vi "HTTPS Server Test with BIO & TCPIP Nodes.vi"() -> ()   [LabVIEW 2013]
uses:
  SSL_Lib/SSL-Lib/Library Paths.ctl
  SSL_Lib/SSL/SSL_Mode.ctl
  SSL_Lib/SSL-Lib/SSL-Lib.lvclass
  SSL_Lib/SSL-Context/SSL-Context.lvclass
  SSL_Lib/SSL/SSL.lvclass
  SSL_Lib/BIO/BIO.lvclass
panel:
  out "Read bytes":string
  out "Numeric":i32
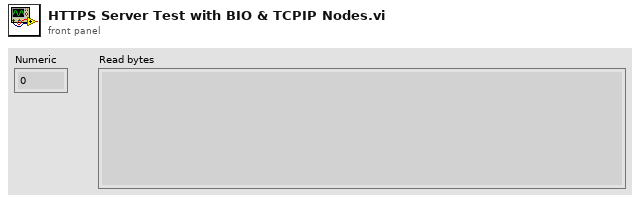
[diagram p1: front panel]
types:
  T1 = typedef "SSL_Lib.lvlib/SSL.lvclass/SSL_Mode.ctl" = i32
  T2 = typedef "SSL_Lib.lvlib/SSL-Lib.lvclass/Library Paths.ctl" = cluster{"SSL Library Path":path, "Crypto Library Path":path}
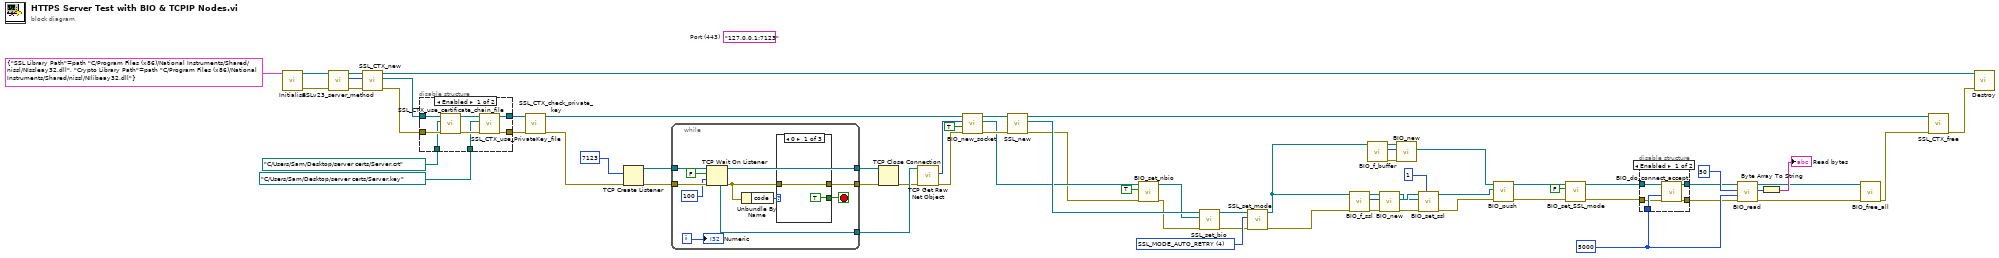
[diagram p0: block diagram]
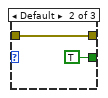
[diagram p3: hidden frame]
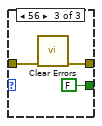
[diagram p4: hidden frame]
diagram:
  w37 = u32 5000 ("Timeout (10000ms)")
  (unwired) "127.0.0.1:7123"  # Port (443)
  w54 = T1 4 items=["None"=0, "SSL_MODE_ENABLE_PARTIAL_WRITE"=1, "SSL_MODE_ACCEPT_MOVING_WRITE_BUFFER"=2, "SSL_MODE_AUTO_RETRY"=4, "SSL_MODE_RELEASE_BUFFERS"=16, "SSL_MODE_SEND_FALLBACK_SCSV"=128] ("Mode")
  n1 = call "Initialise.vi"("Library Paths"=T2 {"SSL Library Path"=path "C:/Program Files (x86)/National Instruments/Shared/nissl/NIssleay32.dll", "Crypto Library Path"=path "C:/Program Files (x86)/National Instruments/Shared/nissl/NIlibeay32.dll"}) -> ("error out"=w63:errorcluster, "SSL-Lib out"=w67:refnum<class "SSL-Lib.lvclass">)  [unwired: 9 in]
  n2 = call "SSLv23_server_method.vi"("error in (no error)"=w63, "SSL-Lib in"=w67) -> ("error out"=w61:errorcluster, "*SSL_Method"=w66:u64, "SSL-Lib out"=w65:refnum<class "SSL-Lib.lvclass">)  [unwired: 7 in]
  n3 = call "SSL_CTX_new.vi"("error in (no error)"=w61, "*SSL_Method"=w66, "SSL-Lib in"=w65) -> ("error out"=w60:errorcluster, "SSL-Context out"=w59:refnum<class "SSL-Context.lvclass">, "SSL-Lib out"=w53:refnum<class "SSL-Lib.lvclass">)  [unwired: 6 in]
  n4 = disable-structure shown="Enabled" {
    disable-tunnel: w60 -> [w73 w76]
    disable-tunnel: w59 -> [w72 w77]
    disable-tunnel: [w71 w76] -> w58
    disable-tunnel: [w70 w77] -> w57
    disable-tunnel: path "C:/Users/Sam/Desktop/server certs/Server.crt" -> [w69 _]
    disable-tunnel: path "C:/Users/Sam/Desktop/server certs/Server.key" -> [w68 _]
    frame Enabled {
      n5 = call "SSL_CTX_use_certificate_chain_file.vi"("error in (no error)"=w73, "Certificate Chain File"=w69, "SSL-Context in"=w72) -> ("error out"=w75:errorcluster, "SSL-Context out"=w74:refnum<class "SSL-Context.lvclass">)  [unwired: 7 in]
      n6 = call "SSL_CTX_use_PrivateKey_file.vi"("error in (no error)"=w75, "PrivateKey File"=w68, "SSL-Context in"=w74) -> ("error out"=w71:errorcluster, "SSL-Context out"=w70:refnum<class "SSL-Context.lvclass">)  [unwired: 7 in]
    }
    frame Disabled {
    }
  }
  n7 = call "SSL_CTX_check_private_key.vi"("error in (no error)"=w58, "SSL-Context in"=w57) -> ("error out"=w45:errorcluster, "SSL-Context out"=w30:refnum<class "SSL-Context.lvclass">)  [unwired: 8 in]
  n8 = TCP Create Listener(8:w45, 10:u16 7123 ("port")) -> (0:w51:errorcluster, 3:w50:refnum<k5>)  [unwired: 3 in, 1 out]
  n9 = while {
    tunnel: w51 -> [w88]
    tunnel: w50 -> [w87]
    tunnel: [w86] -> w49
    tunnel: [w82] -> w48
    tunnel: [w85] -> w47
    i -> [w78]
    stop <- w81 stop-if-true
    n10 = TCP Wait On Listener(8:w88, 9:100 ("timeout ms (wait forever: -1)"), 10:FALSE ("resolve remote address (T)"), 11:w87) -> (0:w83:errorcluster, 3:w86:refnum<k5>, 4:w85:refnum<k5>)  [unwired: 2 out]
    n11 = Unbundle By Name(w83) -> ("code"=w84:i32)
    n12 = case shown="0" w84 {
      tunnel: w83 -> [w90 w92 w95]
      tunnel: [w90 w92 w94] -> w82
      tunnel: [TRUE TRUE FALSE] -> w81
      frame 0 {
      }
      frame Default {
      }
      frame 56 {
        n13 = call <vilib>:"Clear Errors.vi"("error in (no error)"=w95) -> ("error out"=w94:errorcluster)  [unwired: 6 in]
      }
    }
    "Numeric" <- w78
  }
  n14 = TCP Close Connection(connection ID=w49, error in (no error)=w48) -> (error out=w46:errorcluster)  [unwired: 1 in, 1 out]
  n15 = call <vilib>:"TCP Get Raw Net Object.vi"("error in (no error)"=w46, "connection ID"=w47) -> ("error out"=w33:errorcluster, "raw net object"=w32:u64)  [unwired: 7 in, 1 out]
  n16 = call "BIO_new_socket.vi"("error in (no error)"=w33, "Close on free? (T)"=TRUE, "fd"=w32, "SSL-Context in"=w30) -> ("error out"=w29:errorcluster, "Socket BIO out"=w26:refnum<class "BIO.lvclass">, "SSL-Context out"=w28:refnum<class "SSL-Context.lvclass">)  [unwired: 5 in]
  n17 = call "SSL_new.vi"("error in (no error)"=w29, "SSL-Context in"=w28) -> ("error out"=w23:errorcluster, "SSL out"=w27:refnum<class "SSL.lvclass">, "SSL-Context out"=w44:refnum<class "SSL-Context.lvclass">)  [unwired: 7 in]
  n18 = call "BIO_set_nbio.vi"("error in (no error)"=w23, "Non-Blocking?"=TRUE, "BIO in"=w26) -> ("error out"=w22:errorcluster, "BIO out"=w24:refnum<class "BIO.lvclass">)  [unwired: 7 in]
  n19 = call "SSL_set_bio.vi"("error in (no error)"=w22, "BIO"=w24, "SSL in"=w27) -> ("error out"=w21:errorcluster, "SSL out"=w25:refnum<class "SSL.lvclass">)  [unwired: 7 in]
  n20 = call "SSL_set_mode.vi"("error in (no error)"=w21, "Mode"=w54, "SSL in"=w25) -> ("error out"=w12:errorcluster, "SSL out"=w5:refnum<class "SSL.lvclass">)  [unwired: 7 in]
  n21 = call "BIO_f_ssl.vi"("error in (no error)"=w12, "SSL-Lib in"=w5) -> ("error out"=w17:errorcluster, "*BIO_Method"=w15:u64, "SSL-Lib out"=w16:refnum<class "SSL.lvclass">)  [unwired: 7 in]
  n22 = call "BIO_f_buffer.vi"("SSL-Lib in"=w5) -> ("error out"=w20:errorcluster, "*BIO_Method"=w18:u64, "SSL-Lib out"=w19:refnum<class "SSL.lvclass">)  [unwired: 8 in]
  n23 = call "BIO_new.vi"("error in (no error)"=w17, "*BIO_method"=w15, "SSL-Lib in"=w16) -> ("error out"=w14:errorcluster, "BIO out"=w13:refnum<class "BIO.lvclass">, "SSL-Lib out"=w11:refnum<class "SSL.lvclass">)  [unwired: 6 in]
  n24 = call "BIO_new.vi"("error in (no error)"=w20, "*BIO_method"=w18, "SSL-Lib in"=w19) -> ("BIO out"=w9:refnum<class "BIO.lvclass">)  [unwired: 6 in, 2 out]
  n25 = call "BIO_set_ssl.vi"("close flag"=1, "error in (no error)"=w14, "SSL in"=w11, "BIO in"=w13) -> ("error out"=w7:errorcluster, "BIO out"=w8:refnum<class "BIO.lvclass">)  [unwired: 6 in]
  n26 = call "BIO_push.vi"("error in (no error)"=w7, "New BIO"=w8, "BIO in"=w9) -> ("error out"=w6:errorcluster, "BIO out"=w3:refnum<class "BIO.lvclass">)  [unwired: 7 in]
  n27 = call "BIO_set_SSL_mode.vi"("error in (no error)"=w6, "Client?"=FALSE, "BIO in"=w3) -> ("error out"=w4:errorcluster, "BIO out"=w2:refnum<class "BIO.lvclass">)  [unwired: 7 in]
  n28 = disable-structure shown="Enabled" {
    disable-tunnel: w2 -> [w100 w102]
    disable-tunnel: w37 -> [w99 _]
    disable-tunnel: [w98 w102] -> w36
    disable-tunnel: [w97 w101] -> w35
    disable-tunnel: w4 -> [w96 w101]
    frame Enabled {
      n29 = call "BIO_do_connect_accept.vi"("error in (no error)"=w96, "Timeout (10000ms)"=w99, "BIO in"=w100) -> ("error out"=w97:errorcluster, "BIO out"=w98:refnum<class "BIO.lvclass">)  [unwired: 7 in]
    }
    frame Disabled {
    }
  }
  n30 = call "BIO_read.vi"("error in (no error)"=w35, "Timeout (10000ms)"=w37, "bytes to read"=50, "BIO in"=w36) -> ("error out"=w39:errorcluster, "Bytes read"=w41:u8[], "BIO out"=w34:refnum<class "BIO.lvclass">)  [unwired: 5 in]
  n31 = Byte Array To String(unsigned byte array=w41) -> (string=→"Read bytes":string)
  n32 = call "BIO_free_all.vi"("error in (no error)"=w39, "BIO in"=w34) -> ("error out"=w38:errorcluster)  [unwired: 9 in]
  n33 = call "SSL_CTX_free.vi"("error in (no error)"=w38, "SSL-Context in"=w44) -> ("error out"=w62:errorcluster)  [unwired: 9 in]
  n34 = call "Destroy.vi"("error in (no error)"=w62, "SSL-Lib in"=w53) -> ()  [unwired: 9 in, 1 out]
